vi "Read Data from 5772 with DRAM.vi"() -> ()   [LabVIEW 2011]
uses:
  <vilib>/userDefined/High Color/nirio_resource_hc.ctl
  <vilib>/FPGAPlugInAG/PXIe-7965R/niLvFpga_Open_PXIe-7965R.vi
  <vilib>/rvi/interface/common/dynamic/niFpgaDynamicAddResources.vi
  <vilib>/FPGAPlugInAG/Dynamic/niLvFpga_Download_Dynamic.vi
  <vilib>/FPGAPlugInAG/Dynamic/niLvFpga_Run_Dynamic.vi
  <vilib>/Utility/error.llb/Error Cluster From Error Code.vi
  <vilib>/rvi/errors/niLvFpgaAdjustHostInterfaceError.vi
  <vilib>/measure/maspectr.llb/FFT Power Spectrum and PSD for 1 Chan.vi
  <vilib>/FPGAPlugInAG/Dynamic/niLvFpga_Close_Dynamic.vi
  <vilib>/rvi/interface/nirviOpenFPGA/nirviOpenFPGA.xnode
  <userlib>/Fast OCT/Debug/Version 1/FPGA Bitfiles/Current/Acquire 2 channel data with DRAM (fast trig).lvbitx
  <vilib>/rvi/interface/nirviMethod/nirviMethod.xnode
  <vilib>/rvi/interface/nirviReadWriteControl/nirviReadWriteControl.xnode
  <vilib>/rvi/interface/nirviCloseFPGA/nirviCloseFPGA.xnode
  <userlib>/FlexRIO Host Library/FlexRIO Host Library (User).lvlib
  <vilib>/rvi/interface/Simulation/niFpgaSimulationCallBeginRW.vi
  <vilib>/measure/NI_MAPro.lvlib
  <userlib>/FlexRIO Host Library/FlexRIO Host API/Configure/Record Parameters/5772/Configure Record Parameters (5772).vi
  <vilib>/ptbypt/NI_PtbyPt.lvlib
  NiFpgaLv.dll
panel:
  out "Elements Remaining":u32
  out "Host FIFO Timed Out?":bool
  out "Sample Jitter":dbl format="%#_6g Samples"
  out "Phase Shift Histogram":T1(graph)
  out "detected phase (deg)":dbl format="%.2p"
  out "Detected Sine Frequency":dbl format="%.2p"
  out "FFT Size":i32
  out "FFT":cluster{"f0":dbl, "df":dbl, "magnitude":dbl[]}(graph)
  out "Channel 0 Data":i16[][](graph)
  in  "Resource Name":T2="RIO0"
  out "NumSamplesAcquired":u32
  out "Iterations Done":i32
  in  "Stop":bool
  in  "Trigger Type":T3(ring)=enum."Software Trigger"
  in  "Record Count":u32=1
  in  "Pre Trig":u32=16
  in  "Post Trig":u32=16
  out "error out":errorcluster
  # "Gain and Offset\nFrame Trigger"
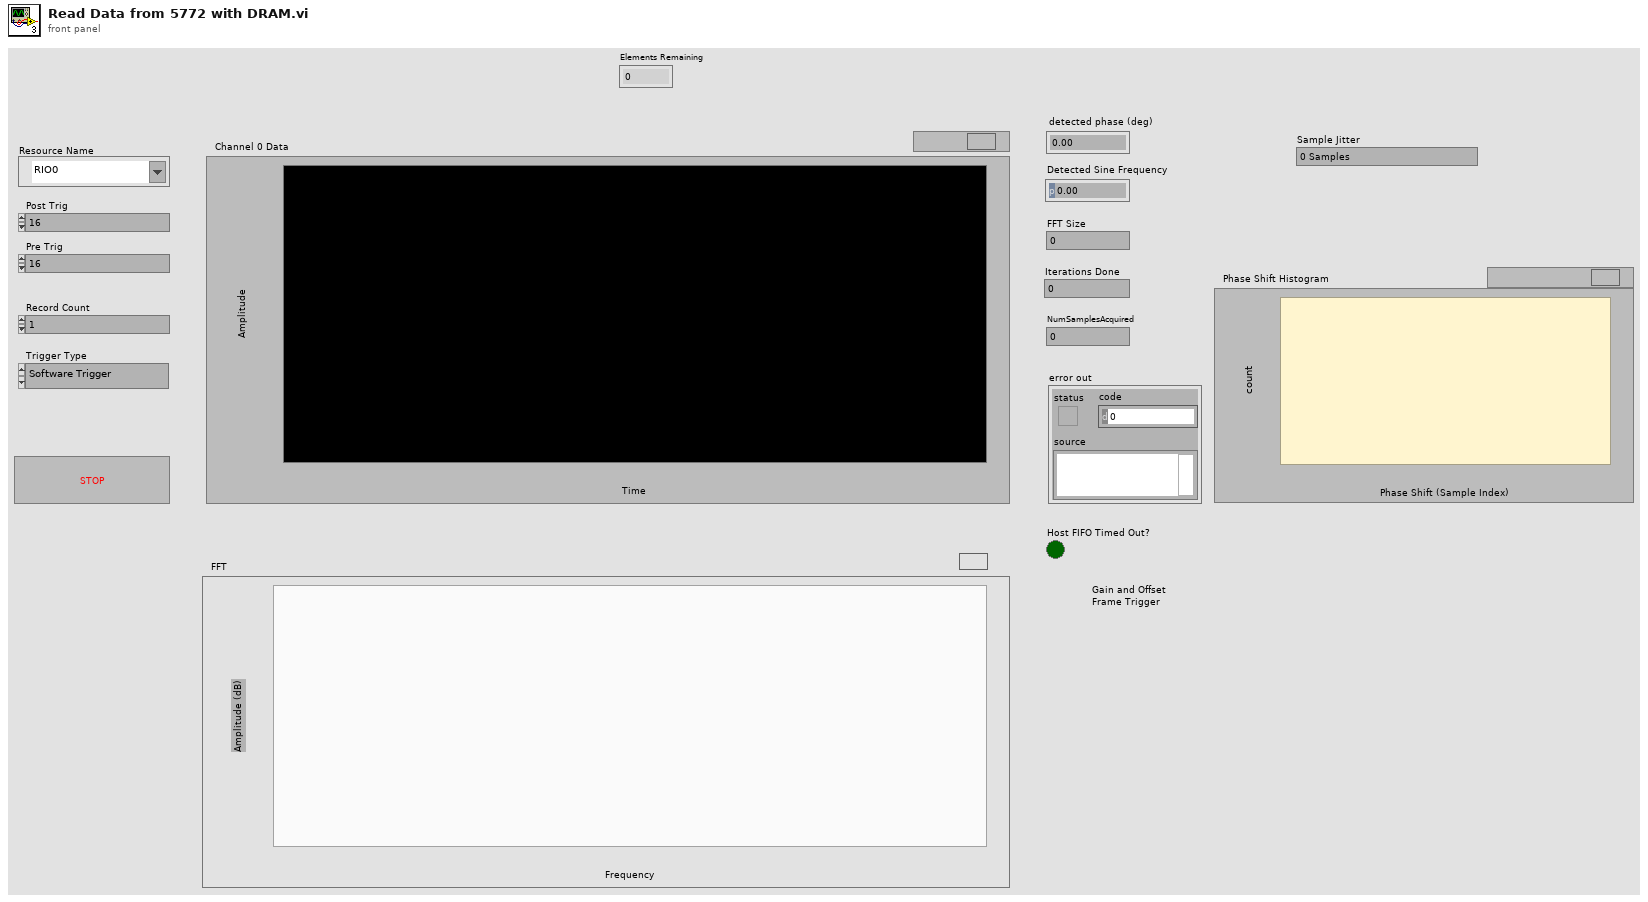
[diagram p1: front panel]
types:
  T1 = cluster{"X Values":dbl[], "Histogram: h(x)":i32[]}
  T2 = typedef "nirio_resource_hc.ctl" = tag
  T3 = enum8{"Immediate Trigger", "Software Trigger", "External Digital Trigger", "Analog Trigger"}
  T4 = cluster{"Load Record Parameters?":bool, "Pre Trigger Samples":u32, "Post Trigger Samples":u32, "Trigger Hold Off":u32, "Record Count":u32}
  T5 = cluster{"write grant time (clocks)":u16, "read grant time (clocks)":u16}
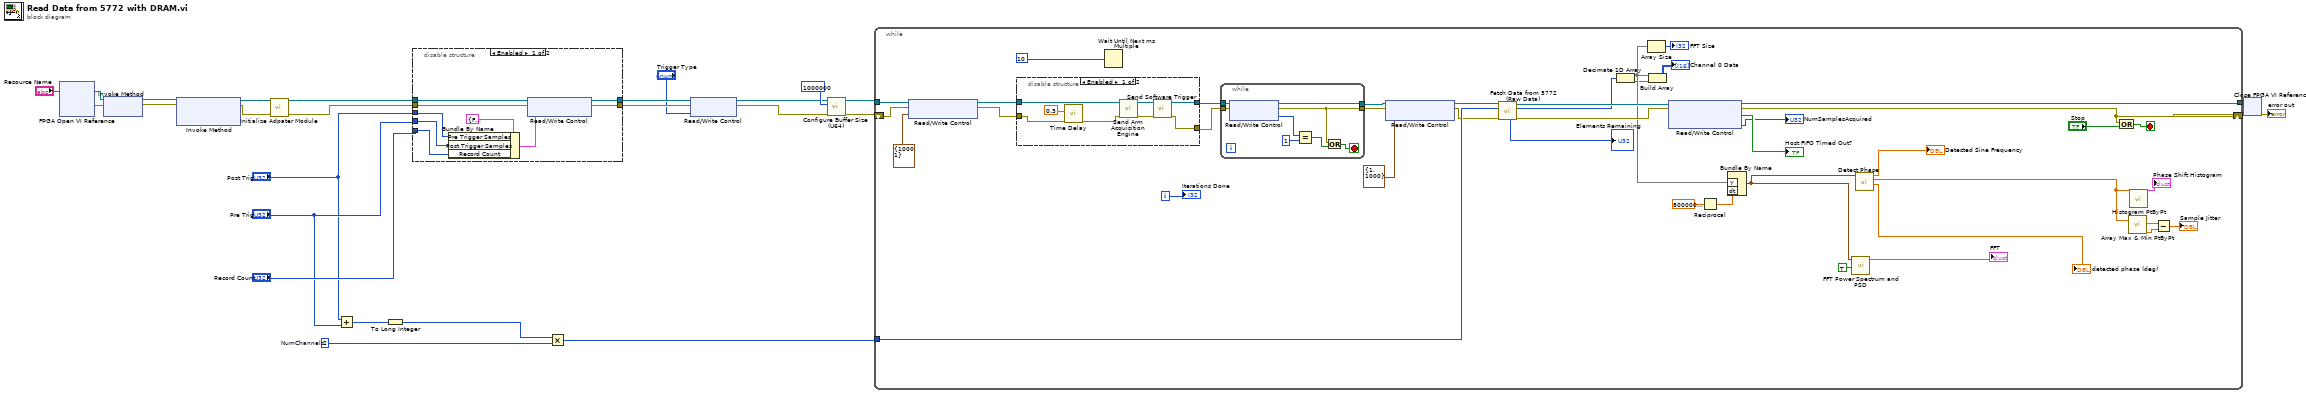
[diagram p0: block diagram]
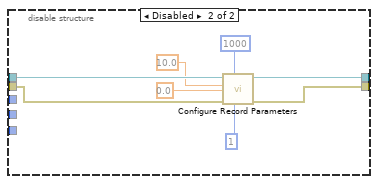
[diagram p2: hidden frame]
diagram:
  w19 = u32 2  # NumChannels
  n1 = xnode "FPGA Open VI Reference"("resource name"="Resource Name") -> ("FPGA VI Reference Out"=w2:refnum<k20>, "error out"=w1:errorcluster)  [unwired: 1 in]
  n2 = xnode "Invoke Method"("FPGA VI Reference In"=w2, "error in"=w1) -> ("FPGA VI Reference Out"=w4:refnum<k20>, "error out"=w3:errorcluster)
  n3 = xnode "Invoke Method"("FPGA VI Reference In"=w4, "error in"=w3) -> ("FPGA VI Reference Out"=w17:refnum<k20>, "error out"=w16:errorcluster)  [unwired: 1 in]
  n4 = call <userlib>:"Initialize Adpater Module.vi"("error in"=w16, "FPGA VI Reference In"=w17) -> ("error out"=w24:errorcluster, "FPGA VI Reference Out"=w25:refnum<k20>)  [unwired: 7 in, 1 out]
  n5 = Add(x="Post Trig", y="Pre Trig") -> (x+y=w9:u32)
  n6 = To Long Integer(number=w9) -> (32bit integer=w5:i32)
  n7 = disable-structure shown="Enabled" {
    disable-tunnel: w25 -> [w36 w45]
    disable-tunnel: w24 -> [w35 w44]
    disable-tunnel: "Record Count" -> [w29 _]
    disable-tunnel: "Pre Trig" -> [w30 _]
    disable-tunnel: [w34 w42] -> w12
    disable-tunnel: [w33 w43] -> w11
    disable-tunnel: "Post Trig" -> [w31 _]
    frame Enabled {
      n8 = Bundle By Name(cluster=T4 {"Load Record Parameters?"=FALSE, "Pre Trigger Samples"=0, "Post Trigger Samples"=0, "Trigger Hold Off"=0, "Record Count"=0} ("Record Parameters"), "Pre Trigger Samples"=w31, "Post Trigger Samples"=w30, "Record Count"=w29) -> (w28:T4)
      n9 = xnode "Read/Write Control"("FPGA VI Reference In"=w36, "error in"=w35, "Record Parameters"=w28) -> ("FPGA VI Reference Out"=w34:refnum<k20>, "error out"=w33:errorcluster)
    }
    frame Disabled {
      n10 = call-poly <userlib>:"Configure Record Parameters.vi"("Record Count"=u16 1, "Record Length"=u16 1000, "error in"=w44, "% of Acquisition Hold Off Time"=0.0, "% of Pre-Trigger Samples"=10.0, "FPGA VI Reference In"=w45) -> ("error out"=w43:errorcluster, "FPGA VI Reference Out"=w42:refnum<k20>, "Actual Record Length"=w39:u16)  [unwired: 3 in]
    }
  }
  n11 = Multiply(x=w5, y=w19) -> (x*y=w18:u32)
  n12 = xnode "Read/Write Control"("FPGA VI Reference In"=w12, "error in"=w11, "Trigger Type"="Trigger Type") -> ("FPGA VI Reference Out"=w6:refnum<k20>, "error out"=w7:errorcluster)
  n13 = call <userlib>:"Configure Buffer Size (U64).vi"("error in"=w7, "Buffer Size"=u32 1000000, "FPGA VI Reference In"=w6) -> ("error out"=w14:errorcluster, "FPGA VI Reference Out"=w15:refnum<k20>)  [unwired: 7 in]
  n14 = while {
    shift-right: [w82] -> w21
    shift-left: w14 -> [w62]
    tunnel: w15 -> [w63]
    tunnel: [w83] -> w22
    tunnel: w18 -> [w73]
    i -> [w51]
    stop <- w85 stop-if-true
    n15 = xnode "Read/Write Control"("FPGA VI Reference In"=w63, "error in"=w62, "DRAM Arbiter Config"=T5 {"write grant time (clocks)"=1000, "read grant time (clocks)"=1}) -> ("FPGA VI Reference Out"=w61:refnum<k20>, "error out"=w60:errorcluster)
    n16 = disable-structure shown="Enabled" {
      disable-tunnel: w61 -> [w102 w104]
      disable-tunnel: w60 -> [w96 w103]
      disable-tunnel: [w98 w104] -> w55
      disable-tunnel: [w99 w103] -> w54
      frame Enabled {
        n17 = call "Time Delay"("error in (no error)"=w96, "Delay Time (s)"=0.3) -> ("error out"=w95:errorcluster)  [unwired: 9 in]
        n18 = call <userlib>:"Send Arm Acquisition Engine.vi"("error in"=w95, "FPGA VI Reference In"=w102) -> ("error out"=w100:errorcluster, "FPGA VI Reference Out"=w101:refnum<k20>)  [unwired: 8 in]
        n19 = call <userlib>:"Send Software Trigger.vi"("error in"=w100, "FPGA VI Reference In"=w101) -> ("error out"=w99:errorcluster, "FPGA VI Reference Out"=w98:refnum<k20>)  [unwired: 8 in]
      }
      frame Disabled {
      }
    }
    n20 = Wait Until Next ms Multiple(millisecond multiple=u32 10) -> ()  [unwired: 1 out]
    n21 = while {
      tunnel: w55 -> [w94]
      tunnel: w54 -> [w93]
      tunnel: [w92] -> w53
      tunnel: [w89] -> w52
      stop <- w88 stop-if-true
      n22 = xnode "Read/Write Control"("FPGA VI Reference In"=w94, "error in"=w93) -> ("FPGA VI Reference Out"=w92:refnum<k20>, "error out"=w89:errorcluster, "Record Count"=w91:u32)
      n23 = Equal?(x=w91, y=u32 1) -> (x = y?=w90:bool)
      n24 = Or(x=w89, y=w90) -> (x .or. y?=w88:bool)
    }
    n25 = xnode "Read/Write Control"("FPGA VI Reference In"=w53, "error in"=w52, "DRAM Arbiter Config"=T5 {"write grant time (clocks)"=1, "read grant time (clocks)"=1000}) -> ("FPGA VI Reference Out"=w58:refnum<k20>, "error out"=w57:errorcluster)
    n26 = call <userlib>:"Fetch Data from 5772 (Raw Data).vi"("error in"=w57, "Samples"=w73, "FPGA VI Reference In"=w58) -> ("error out"=w80:errorcluster, "Data Acquired"=w66:i16[], "FPGA VI Reference Out"=w81:refnum<k20>, "Elements Remaining"=→"Elements Remaining":u32)  [unwired: 5 in]
    n27 = Decimate 1D Array(w66) -> (w48:i16[], w47:i16[])
    n28 = Array Size(array=w48) -> (size(s)=→"FFT Size":i32)
    n29 = Build Array(w48, w47) -> (→"Channel 0 Data":i16[][])
    n30 = xnode "Read/Write Control"("FPGA VI Reference In"=w81, "error in"=w80) -> ("FPGA VI Reference Out"=w83:refnum<k20>, "error out"=w82:errorcluster, "Host FIFO Timed Out?"=→"Host FIFO Timed Out?":bool, "U256s Acquired"=→"NumSamplesAcquired":u32)
    n31 = Reciprocal(x=800000000.0) -> (1/x=w78:dbl)
    n32 = Bundle By Name("Y"=w48, "dt"=w78) -> (w74:waveform(i16))  [unwired: 1 in]
    n33 = call-poly <vilib>:"FFT Power Spectrum and PSD.vi"("dB On (F)"=TRUE, "time signal"=w74) -> ("Power Spectrum / PSD"=→"FFT":cluster{"f0":dbl, "df":dbl, "magnitude":dbl[]})  [unwired: 6 in, 3 out]
    n34 = call <userlib>:"Detect Phase.vi"("Input Wavceform"=w74) -> ("Phase in Degress"=→"detected phase (deg)":dbl, "Phase in Samples"=w67:dbl, "Detected Sine Frequency"=→"Detected Sine Frequency":dbl)  [unwired: 8 in]
    n35 = Compound Arithmetic op=OR(w82, "Stop") -> (w85:bool)
    n36 = call <vilib>:"Array Max & Min PtByPt.vi"("input data point"=w67) -> ("max value"=w71:dbl, "min value"=w70:dbl)  [unwired: 2 in, 3 out]
    n37 = call <vilib>:"Histogram PtByPt.vi"("x"=w67) -> ("Histogram Graph"=→"Phase Shift Histogram":T1)  [unwired: 7 in, 3 out]
    n38 = Subtract(x=w71, y=w70) -> (x-y=→"Sample Jitter":dbl)
    "Iterations Done" <- w51
  }
  n39 = xnode "Close FPGA VI Reference"("FPGA VI Reference In"=w22, "error in"=w21) -> ("error out"=→"error out":errorcluster)
